vi "Byte Array to Numeric.vi"(1 "2 Bytes":u8[](array[numeric]) format="%x") -> (0 "U16 Numba":u16)   [LabVIEW 2016]
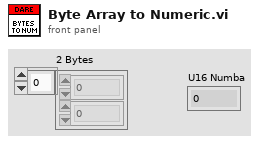
[diagram p1: front panel]
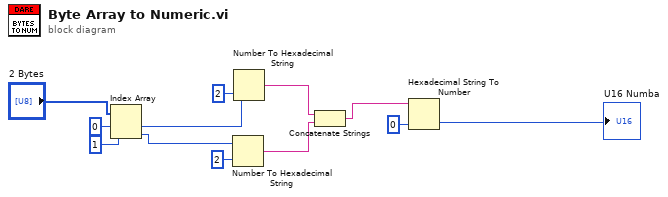
[diagram p0: block diagram]
diagram:
  n1 = Index Array(array="2 Bytes", index #1=0 ("index"), index #2=1 ("index")) -> (element #1=w9:u8, element #2=w6:u8)
  n2 = Number To Hexadecimal String(1:i16 2 ("width (-)"), 2:w6) -> (0:w4:string)
  n3 = Number To Hexadecimal String(1:i16 2 ("width (-)"), 2:w9) -> (0:w5:string)
  n4 = Concatenate Strings(w5, w4) -> (w3:string)
  n5 = Hexadecimal String To Number(string=w3, default (0uL)=u16 0 ("default (0 U32)")) -> (number=→"U16 Numba":u16)  [unwired: 1 in, 1 out]
